vi "st_str Main.vi"() -> ()   [LabVIEW 2017]
doc: "This sample project is........"
uses:
  controls/st_str State.ctl
  controls/st_str Data.ctl
  controls/st_str UI References.ctl
  controls/st_str Graph Data.ctl
  <vilib>/Utility/miscctls.llb/LVAnnotationListTypeDef.ctl
  <vilib>/Utility/miscctls.llb/LVCursorListTypeDef.ctl
  controls/st_str User Specified Data.ctl
  controls/st_str HW Configuration.ctl
  controls/st_str Simulated Signal Type.ctl
  controls/st_str Analysis Configuration.ctl
  controls/st_str New Data Behavior.ctl
  st_voltmetr/subVIs/st_str Global.vi
  subVIs/st_str Settings Dialog(VIForIzm).vi
panel:
  in  "FirstActiveParam":bool
  out "АЧХ 2":cluster{dbl[], dbl[]}[](graph) caption="XY Graph - Light"
  in  "SetParametrsGen":bool
  out "Connect\nVoltmetr":bool
  in  "TypeGraph":T1(radio)
  in  "ResultTbl":string[][](table)
  out "Graph":waveform(dbl)[](graph)
  in  "Start":bool
  in  "View":enum16{"График", "Таблица"}(ring)
  in  "Open":bool
  in  "Delete":bool
  in  "Report":bool
  in  "Save":bool
  in  "Settings":bool
  in  "Snapshot":bool
  in  "Analyze":bool
  in  "Clear":bool
  in  "Exit":bool
  in  "Acquire":bool
  in  "Export":bool
  in  "Save Data":bool
  in  "Load Data":bool
  out "Status Bar":string
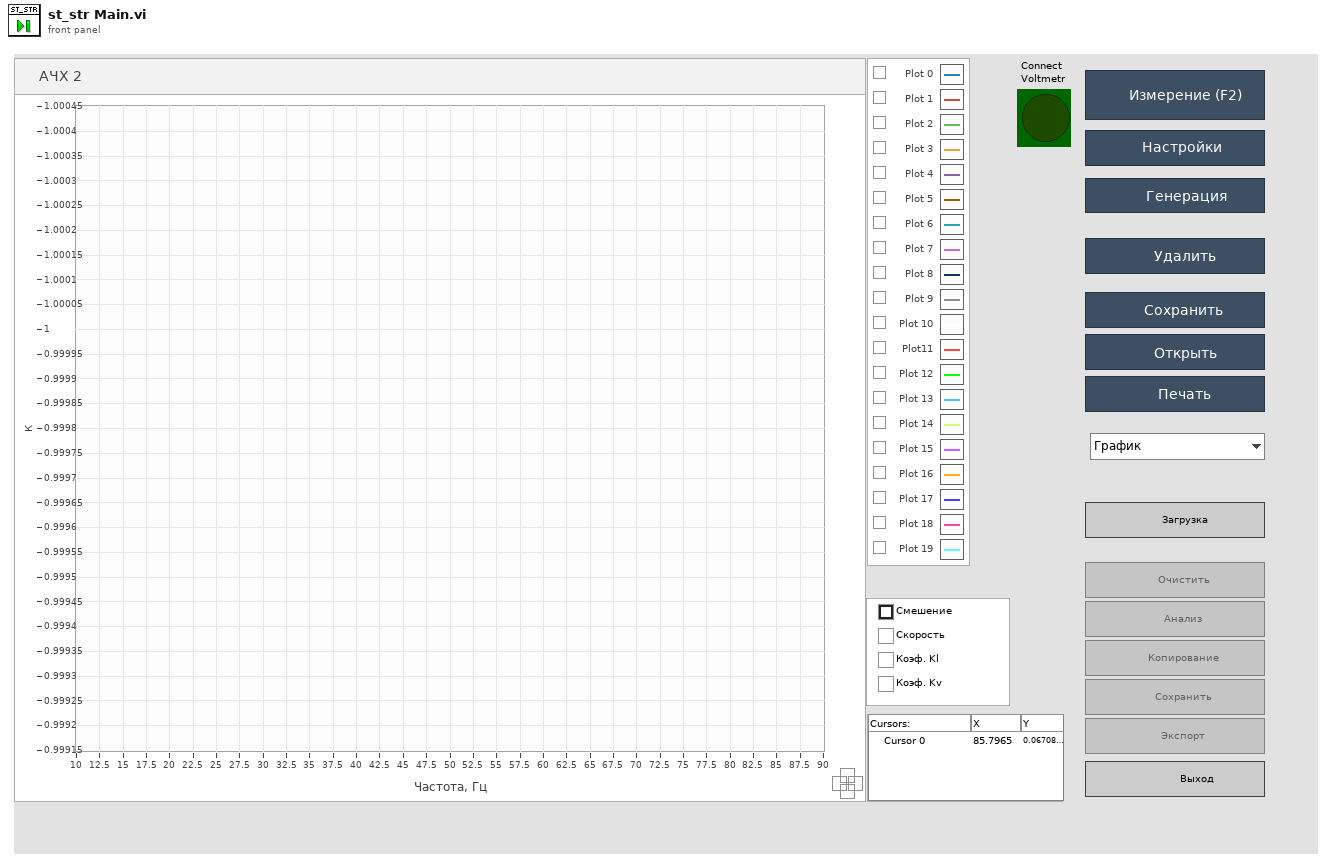
[diagram p1: front panel]
types:
  T1 = enum32{"Смешение", "Скорость", "Коэф. Kl", "Коэф. Kv"}
  T2 = typedef "st_str Data.ctl" = cluster{"UI References":T3, "Graph Data":T4, "User Specified":T7, "GenParametr":cluster{"UgenVrms":dbl, "Frequency 1,kHz":dbl, "dFreq, kHz":dbl, "Frequency 2,kHz":dbl, "WaitSignalGen":dbl}}
  T3 = typedef "st_str UI References.ctl" = cluster{"Exit Ref":refnum<vi>, "Save Ref":refnum<vi>, "Open Ref":refnum<vi>, "Export Ref":refnum<vi>, "Acquire Ref":refnum<vi>, "Configure Ref":refnum<vi>, "Graph Ref":refnum<vi>, "Clear Ref":refnum<vi>, "Analyze Ref":refnum<vi>, "Status Ref":refnum<vi>, "Snapshot Ref":refnum<vi>, "Tbl Ref":refnum<vi>, "XYGraph Ref":refnum<vi>}
  T4 = typedef "st_str Graph Data.ctl" = cluster{"Data":waveform(dbl)[], "Annotation List":T5, "Cursor List":T6, "Analysis Data":waveform(dbl)[], "XY graph":cluster{"X":dbl[], "Y":dbl[]}[]}
  T5 = typedef "LVAnnotationListTypeDef.ctl" = cluster{"Name":string, "Color":u32, "Style":u8, "Point Style":u8, "Name Visible":bool, "Allow Drag":bool, "Annotation Mode":u32, "Plot":i32, "Index":i32, "Position":cluster{"X":dbl, "Y":dbl}, "X Scale":u32, "Y Scale":u32, "Show Arrow":bool, "Lock Name":bool, "Plot Area":i32, "Label Offset":cluster{"X":dbl, "Y":dbl}}[]
  T6 = typedef "LVCursorListTypeDef.ctl" = cluster{"Name":string, "Color":u32, "Style":u8, "Point Style":u8, "Name Visible":bool, "Allow Drag":bool, "Cursor Mode":u32, "Plot":i32, "Index":i32, "Position":cluster{"X":dbl, "Y":dbl}, "X Scale":u32, "Y Scale":u32, "Watch Plots":i32[], "Watch All Plots":bool, "Plot Area":i32, "Label Offset":cluster{"X":dbl, "Y":dbl}}[]
  T7 = typedef "st_str User Specified Data.ctl" = cluster{"Hardware Configuration":T8, "Analysis Configuration":T10, "New Data Behavior":T11}
  T8 = typedef "st_str HW Configuration.ctl" = cluster{"HW Refnum <Replace Me>":string, "Signal Type <Replace Me>":T9}
  T9 = typedef "st_str Simulated Signal Type.ctl" = enum16{"Sine Wave", "Square Wave"}
  T10 = typedef "st_str Analysis Configuration.ctl" = cluster{"Statistics":bool}
  T11 = typedef "st_str New Data Behavior.ctl" = enum16{"Replace", "Overlay", "Append"}
  T12 = typedef "st_str State.ctl" = enum16{"View", "Initialize", "Wait for Event", "Update UI", "Configure", "Acquire", "Load Data", "Save Data", "Clear Data", "Export Data", "Analyze", "Copy Graph", "Exit", "Connecting"}
  T13 = cluster{"UgenVrms":dbl, "Frequency 1,kHz":dbl, "dFreq, kHz":dbl, "Frequency 2,kHz":dbl, "WaitSignalGen":dbl}
  T14 = typedef "st_str gen parametr.ctl" = cluster{"UgenVrms":dbl, "Frequency 1,kHz":dbl, "dFreq, kHz":dbl, "Frequency 2,kHz":dbl, "WaitSignalGen":dbl}
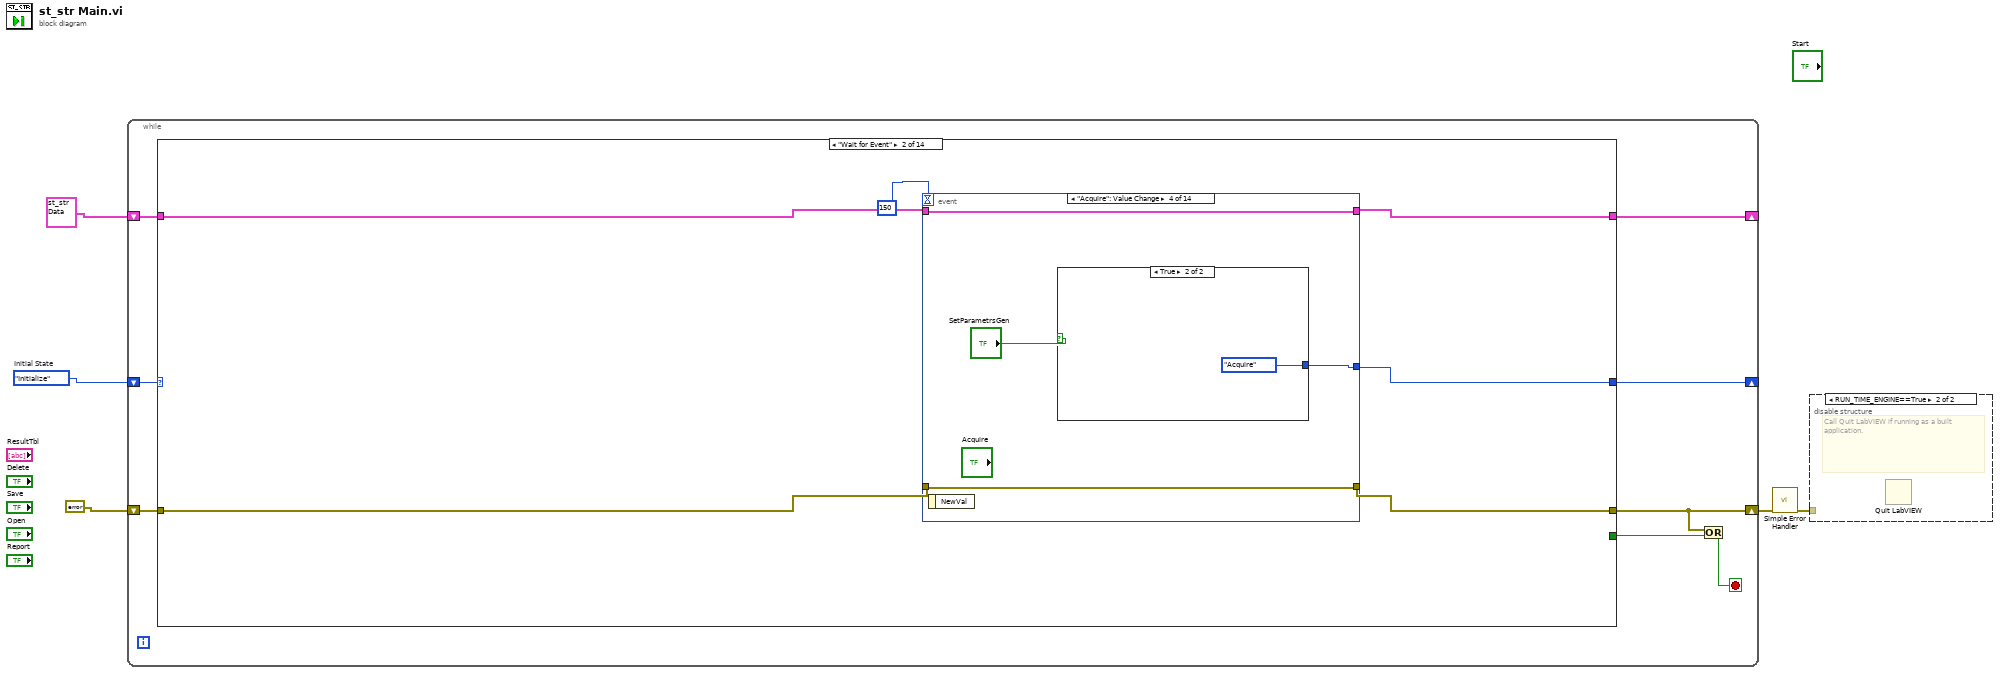
[diagram p0: block diagram]
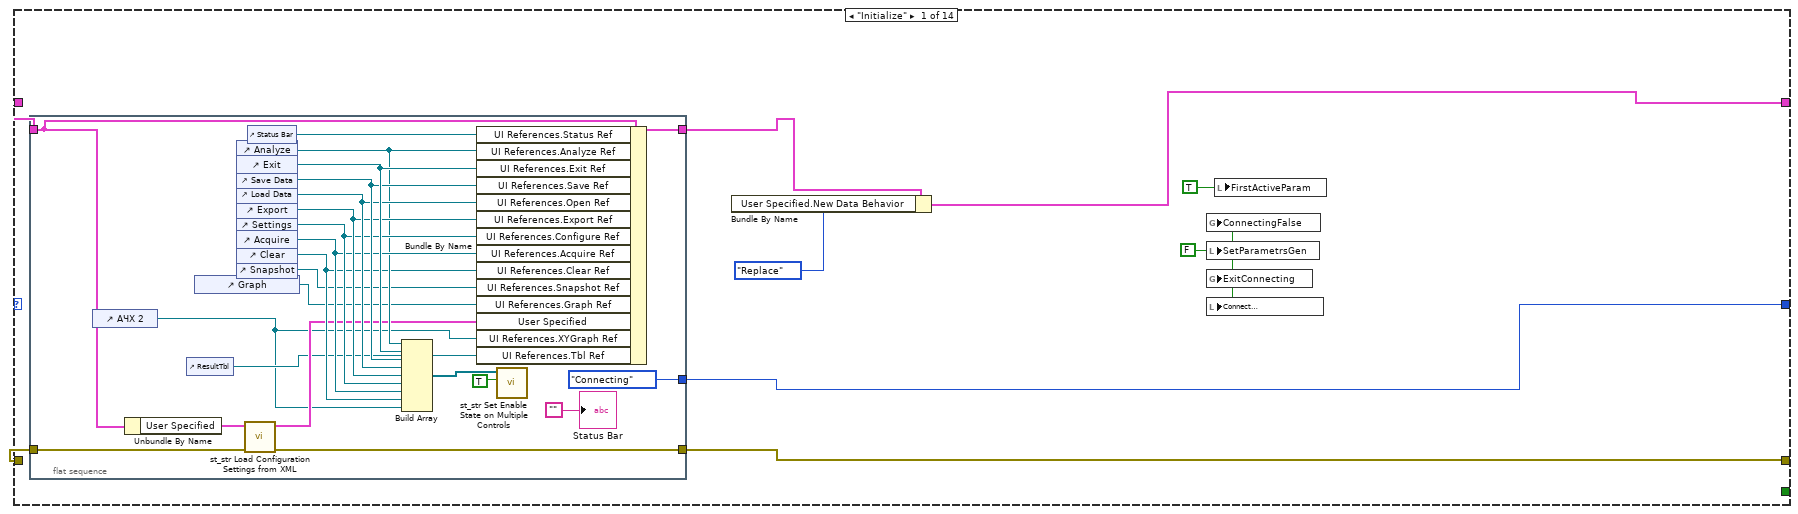
[diagram p3: hidden frame]
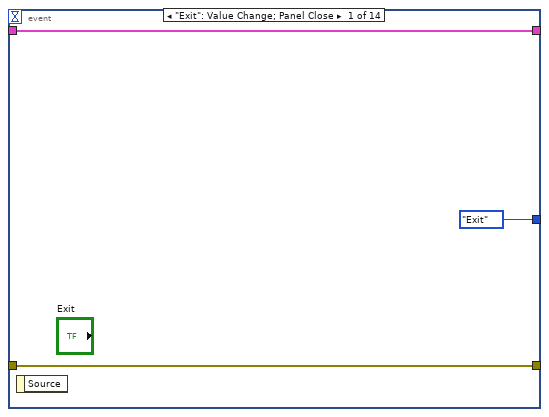
[diagram p4: hidden frame]
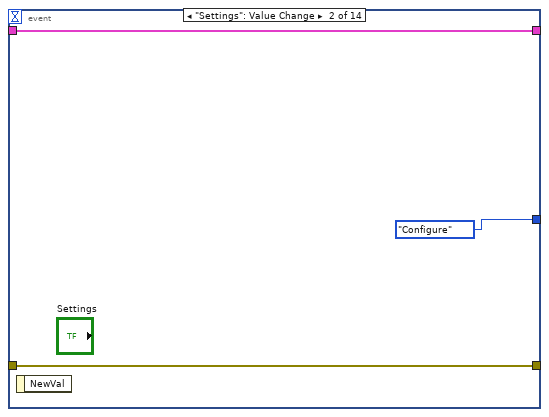
[diagram p5: hidden frame]
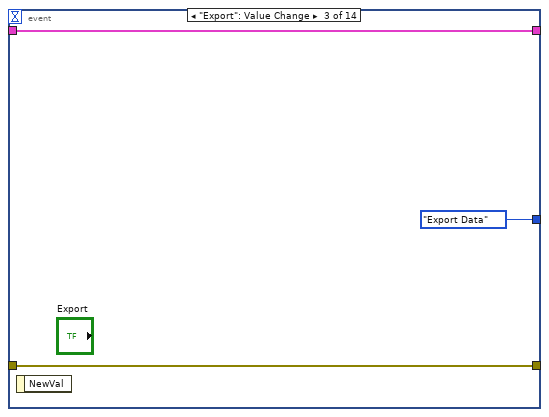
[diagram p6: hidden frame]
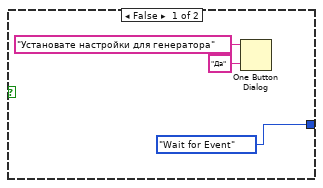
[diagram p7: hidden frame]
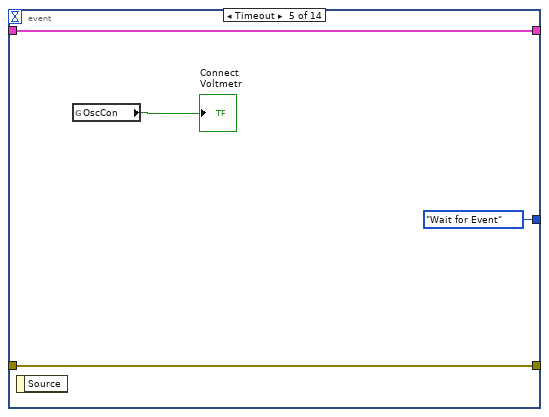
[diagram p8: hidden frame]
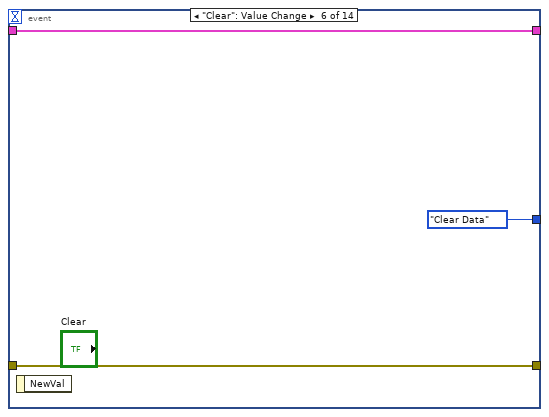
[diagram p9: hidden frame]
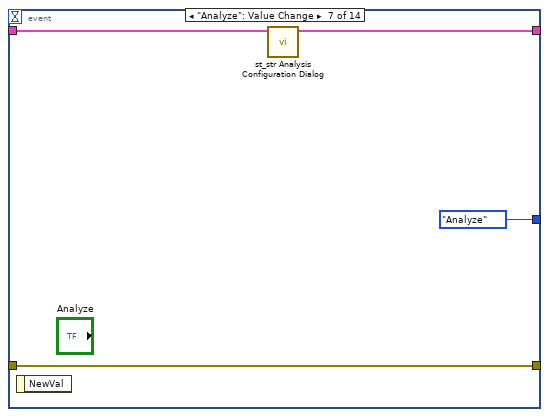
[diagram p10: hidden frame]
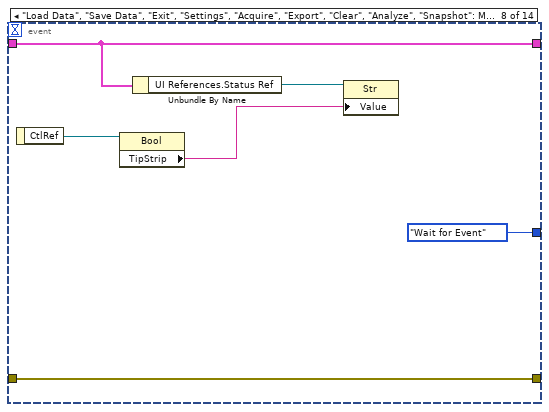
[diagram p11: hidden frame]
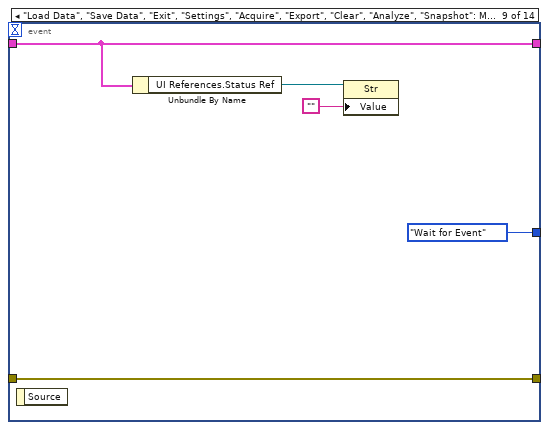
[diagram p12: hidden frame]
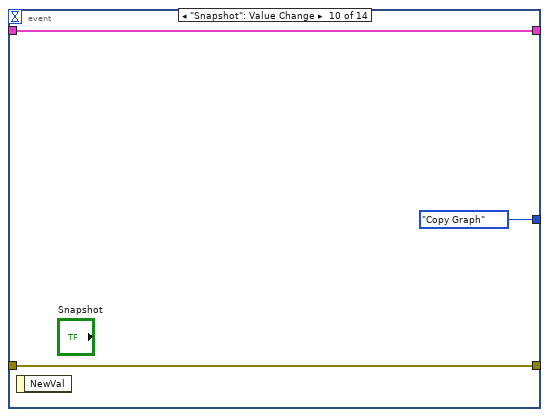
[diagram p13: hidden frame]
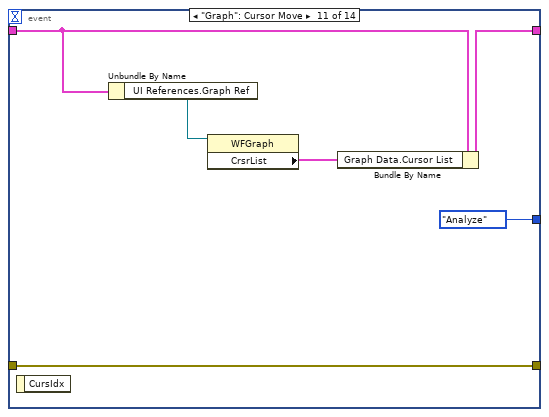
[diagram p14: hidden frame]
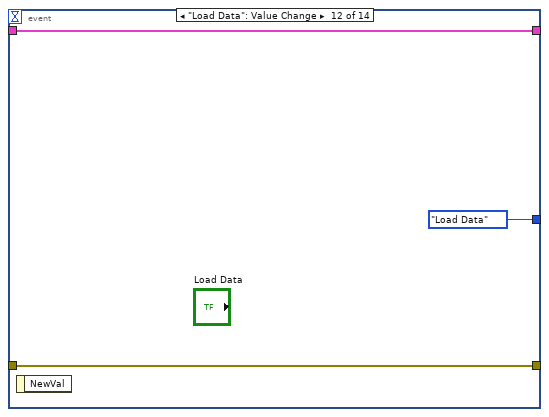
[diagram p15: hidden frame]
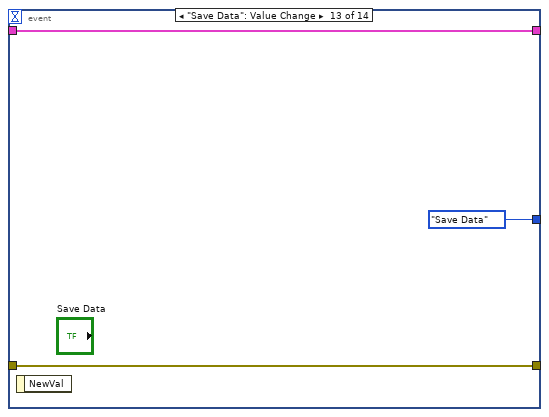
[diagram p16: hidden frame]
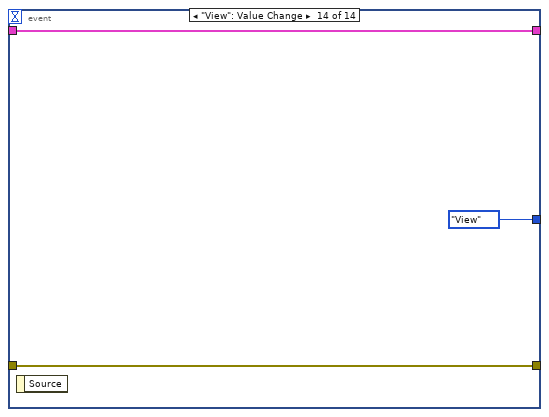
[diagram p17: hidden frame]
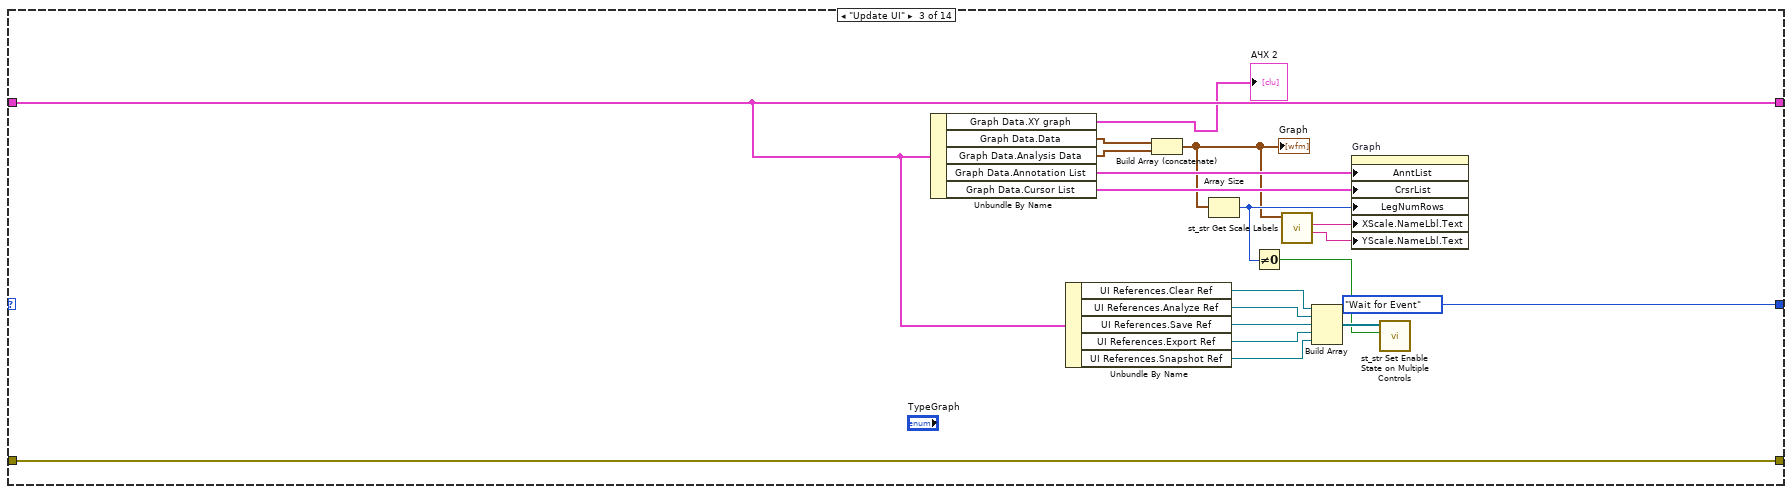
[diagram p18: hidden frame]
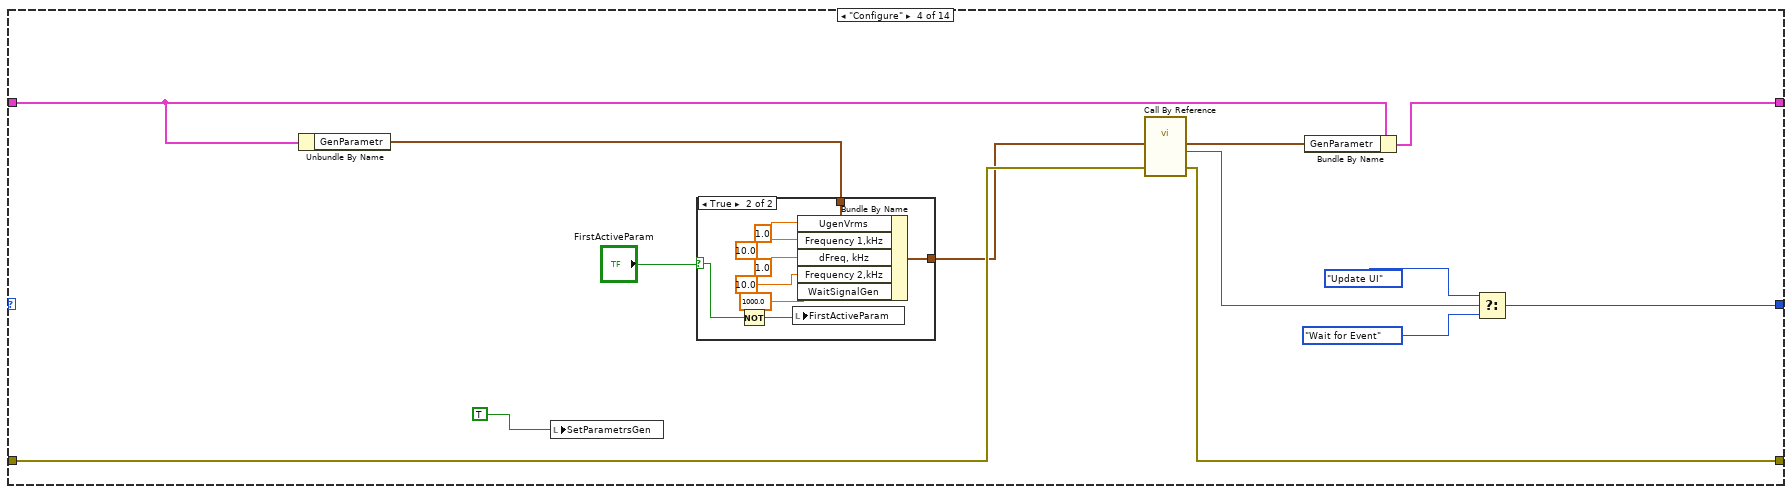
[diagram p19: hidden frame]
diagram:
  w5 = st_str_State."Initialize"  # Initial State
  n1 = while {
    shift-right: [w13] -> _
    shift-left: w5 -> [w6]
    shift-right: [w11] -> _
    shift-left: T2 {"UI References"={"Exit Ref"=refnum, "Save Ref"=refnum, "Open Ref"=refnum, "Export Ref"=refnum, "Acquire Ref"=refnum, "Configure Ref"=refnum, "Graph Ref"=refnum, "Clear Ref"=refnum, "Analyze Ref"=refnum, "Status Ref"=refnum, "Snapshot Ref"=refnum, "Tbl Ref"=refnum, "XYGraph Ref"=refnum}, "Graph Data"={"Data"=[], "Annotation List"=[], "Cursor List"=[], "Analysis Data"=[], "XY graph"=[]}, "User Specified"={"Hardware Configuration"={"HW Refnum <Replace Me>"="", "Signal Type <Replace Me>"=enum."Sine Wave"}, "Analysis Configuration"={"Statistics"=TRUE}, "New Data Behavior"=enum."Replace"}, "GenParametr"={"UgenVrms"=0.0, "Frequency 1,kHz"=0.0, "dFreq, kHz"=0.0, "Frequency 2,kHz"=0.0, "WaitSignalGen"=0.0}} ("Data") -> [w12]
    shift-right: [w7] -> w3
    shift-left: errorcluster {"status"=FALSE, "code"=0, "source"=""} ("error constant") -> [w10]
    stop <- w8 stop-if-true
    # "Finite Measurement State Machine"
    n2 = case shown="\"Wait for Event\"" w6 {
      tunnel: [w22 w51 st_str_State."Wait for Event" ("(Value Not Used)") w134 st_str_State."Update UI" ("Next State") st_str_State."Update UI" ("(Value Not Used)") st_str_State."Wait for Event" ("(Value Not Used)") st_str_State."Wait for Event" ("(Value Not Used)") st_str_State."Update UI" ("(Value Not Used)") st_str_State."Update UI" ("(Value Not Used)") st_str_State."Wait for Event" ("(Value Not Used)") w236 st_str_State."Update UI" ("(Value Not Used)") st_str_State."Update UI" ("(Value Not Used)")] -> w13
      tunnel: [_ _ _ _ _ _ _ _ _ _ _ w235 _ _] -> w9
      tunnel: w12 -> [w21 w50 w110 w140 w161 w182 w195 w207 w218 w221 w227 w233 w243 w260]
      tunnel: [w14 w49 w110 w139 w160 w176 w195 w207 w217 w221 w227 w233 w243 w260] -> w11
      tunnel: w10 -> [w20 w48 w127 w138 w155 w181 w197 w210 w220 w222 w226 w230 w247 w259]
      tunnel: [w19 w47 w127 w137 w158 w180 w193 w204 w220 w222 w225 w229 w247 w259] -> w7
      frame "Initialize" {
        w18 = FALSE ("Connect\nVoltmetr")
        n3 = flat-sequence {
          tunnel: [st_str_State."Connecting" ("Next State")] -> w22
          tunnel: [w44] -> w16
          tunnel: [w33] -> w19
          tunnel: w21 -> [w36]
          tunnel: w20 -> [w34]
          frame #0 {
            n4 = control-ref of="АЧХ 2"() -> (w23:refnum<vi>)
            n5 = Unbundle By Name(w36) -> ("User Specified"=w35:T7)
            n6 = control-ref of="ResultTbl"() -> (w24:refnum<vi>)
            n7 = control-ref of="Graph"() -> (w25:refnum<vi>)
            n8 = control-ref of="Analyze"() -> (w32:refnum<vi>)
            n9 = control-ref of="Exit"() -> (w43:refnum<vi>)
            n10 = control-ref of="Save Data"() -> (w42:refnum<vi>)
            n11 = control-ref of="Load Data"() -> (w41:refnum<vi>)
            n12 = control-ref of="Export"() -> (w40:refnum<vi>)
            n13 = control-ref of="Settings"() -> (w39:refnum<vi>)
            n14 = control-ref of="Acquire"() -> (w38:refnum<vi>)
            n15 = control-ref of="Clear"() -> (w30:refnum<vi>)
            n16 = control-ref of="Snapshot"() -> (w26:refnum<vi>)
            n17 = call "st_str Load Configuration Settings from XML.vi"("error in (no error)"=w34, "User Configuration in"=w35) -> ("error out"=w33:errorcluster, "User Configuration out"=w28:T7)  [unwired: 8 in]
            n18 = control-ref of="Status Bar"() -> (w31:refnum<vi>)
            n19 = Build Array(w32, w43, w42, w41, w40, w39, w38, w30, w23) -> (w37:refnum<vi>[])
            n20 = Bundle By Name(cluster=w36, "UI References.Status Ref"=w31, "UI References.Analyze Ref"=w32, "UI References.Exit Ref"=w43, "UI References.Save Ref"=w42, "UI References.Open Ref"=w41, "UI References.Export Ref"=w40, "UI References.Configure Ref"=w39, "UI References.Acquire Ref"=w38, "UI References.Clear Ref"=w30, "UI References.Snapshot Ref"=w26, "UI References.Graph Ref"=w25, "User Specified"=w28, "UI References.XYGraph Ref"=w23, "UI References.Tbl Ref"=w24) -> (w44:T2)
            n21 = call "st_str Set Enable State on Multiple Controls.vi"("Enable?"=TRUE, "Controls"=w37) -> ()  [unwired: 10 in]
            "Status Bar" <- "" ("Status Bar")
          }
        }
        n22 = Bundle By Name(cluster=w16, "User Specified.New Data Behavior"=st_str_New_Data_Behavior."Replace") -> (w14:T2)
        n23 = global write "st_str Global.vi" "ConnectingFalse"(w18) -> ()
        n24 = local write "SetParametrsGen"(w18) -> ()
        n25 = global write "st_str Global.vi" "ExitConnecting"(w18) -> ()
        n26 = local write "Connect\nVoltmetr"(w18) -> ()
        n27 = local write "FirstActiveParam"(TRUE ("FirstActiveParam")) -> ()
      }
      frame "Wait for Event" {
        n28 = event shown="[3] \"Acquire\": Value Change" {
          selector: _ -> [_ _ _ _ _ _ _ _ _ _ _ _ _ _]
          dyn-events: _ -> [_ _ _ _ _ _ _ _ _ _ _ _ _ _]
          timeout: 150 -> [_ _ _ _ _ _ _ _ _ _ _ _ _ _]
          tunnel: [st_str_State."Exit" ("Next State") st_str_State."Configure" ("Next State") st_str_State."Export Data" ("Next State") w62 st_str_State."Wait for Event" ("Next State") st_str_State."Clear Data" ("Next State") st_str_State."Analyze" ("Next State") st_str_State."Wait for Event" ("Next State") st_str_State."Wait for Event" ("Next State") st_str_State."Copy Graph" ("Next State") st_str_State."Analyze" ("Next State") st_str_State."Load Data" ("Next State") st_str_State."Save Data" ("Next State") st_str_State."View" ("Next State")] -> w51
          tunnel: w50 -> [w53 w57 w60 w64 w72 w75 w77 w83 w89 w93 w94 w101 w104 w108]
          tunnel: [w53 w57 w60 w64 w72 w75 w76 w83 w89 w93 w97 w101 w104 w108] -> w49
          tunnel: w48 -> [w52 w56 w59 w63 w71 w74 w79 w85 w90 w92 w99 w100 w103 w107]
          tunnel: [w52 w56 w59 w63 w71 w74 w79 w85 w90 w92 w99 w100 w103 w107] -> w47
          event "Exit": Value Change; Panel Close {
            n29 = event-data() -> ()  [unwired: 1 in, 1 out]
          }
          event "Settings": Value Change {
            n30 = event-data() -> ()  [unwired: 1 in, 1 out]
          }
          event "Export": Value Change {
            n31 = event-data() -> ()  [unwired: 1 in, 1 out]
          }
          event "Acquire": Value Change {
            n32 = event-data() -> ()  [unwired: 1 in, 1 out]
            n33 = case shown="True" "SetParametrsGen" {
              tunnel: [st_str_State."Wait for Event" ("Next State") st_str_State."Acquire" ("Next State")] -> w62
              frame False {
                n34 = One Button Dialog(message="Установате настройки для генератора", button name ("OK")="Да") -> ()  [unwired: 1 out]
              }
              frame True {
              }
            }
          }
          event Timeout {
            n35 = event-data() -> ()  [unwired: 1 in, 1 out]
            n36 = global read "st_str Global.vi" "OscCon"() -> (→"Connect\nVoltmetr":bool)
          }
          event "Clear": Value Change {
            n37 = event-data() -> ()  [unwired: 1 in, 1 out]
          }
          event "Analyze": Value Change {
            n38 = event-data() -> ()  [unwired: 1 in, 1 out]
            n39 = call "st_str Analysis Configuration Dialog.vi"("Data in"=w77) -> ("Data out"=w76:T2)  [unwired: 10 in]
          }
          event "Load Data", "Save Data", "Exit", "Settings", "Acquire", "Export", "Clear", "Analyze", "Snapshot": Mouse Enter {
            n40 = event-data() -> ("CtlRef"=w84:refnum<vi>)  [unwired: 1 in]
            n41 = property class="Bool"(reference=w84) -> ("TipStrip"=w81:string)  [unwired: 1 in, 2 out]
            n42 = Unbundle By Name(w83) -> ("UI References.Status Ref"=w82:refnum<vi>)
            n43 = property class="Str"(reference=w82, "Value"=w81) -> ()  [unwired: 1 in, 2 out]
          }
          event "Load Data", "Save Data", "Exit", "Settings", "Acquire", "Export", "Clear", "Analyze", "Snapshot": Mouse Leave {
            n44 = event-data() -> ()  [unwired: 1 in, 1 out]
            n45 = Unbundle By Name(w89) -> ("UI References.Status Ref"=w88:refnum<vi>)
            n46 = property class="Str"(reference=w88, "Value"="") -> ()  [unwired: 1 in, 2 out]
          }
          event "Snapshot": Value Change {
            n47 = event-data() -> ()  [unwired: 1 in, 1 out]
          }
          event "Graph": Cursor Move {
            n48 = event-data() -> ()  [unwired: 1 in, 1 out]
            n49 = Unbundle By Name(w94) -> ("UI References.Graph Ref"=w96:refnum<vi>)
            n50 = property class="WFGraph"(reference=w96) -> ("CrsrList"=w95:T6)  [unwired: 1 in, 2 out]
            n51 = Bundle By Name(cluster=w94, "Graph Data.Cursor List"=w95) -> (w97:T2)
          }
          event "Load Data": Value Change {
            n52 = event-data() -> ()  [unwired: 1 in, 1 out]
          }
          event "Save Data": Value Change {
            n53 = event-data() -> ()  [unwired: 1 in, 1 out]
          }
          event "View": Value Change {
            n54 = event-data() -> ()  [unwired: 1 in, 1 out]
          }
        }
      }
      frame "Update UI" {
        n55 = Unbundle By Name(w110) -> ("Graph Data.XY graph"=→"АЧХ 2":cluster{"X":dbl[], "Y":dbl[]}[], "Graph Data.Data"=w121:waveform(dbl)[], "Graph Data.Analysis Data"=w111:waveform(dbl)[], "Graph Data.Annotation List"=w125:T5, "Graph Data.Cursor List"=w122:T6)
        n56 = Unbundle By Name(w110) -> ("UI References.Clear Ref"=w117:refnum<vi>, "UI References.Analyze Ref"=w116:refnum<vi>, "UI References.Save Ref"=w124:refnum<vi>, "UI References.Export Ref"=w114:refnum<vi>, "UI References.Snapshot Ref"=w115:refnum<vi>)
        n57 = Build Array (concatenate)(w121, w111) -> (w119:waveform(dbl)[])
        "Graph" <- w119
        n58 = Array Size(array=w119) -> (size(s)=w120:i32)
        n59 = Not Equal To 0?(x=w120) -> (x != 0?=w118:bool)
        n60 = call "st_str Get Scale Labels.vi"("Array of Waveforms"=w119) -> ("Y Scale Label Text"=w112:string, "X Scale Label Text"=w113:string)  [unwired: 9 in]
        n61 = Build Array(w117, w116, w124, w114, w115) -> (w123:refnum<vi>[])
        n62 = property on="Graph" class="WFGraph (strict)"("AnntList"=w125, "CrsrList"=w122, "LegNumRows"=w120, "XScale.NameLbl.Text"=w113, "YScale.NameLbl.Text"=w112) -> ()  [unwired: 2 in, 2 out]
        n63 = call "st_str Set Enable State on Multiple Controls.vi"("Enable?"=w118, "Controls"=w123) -> ()  [unwired: 10 in]
      }
      frame "Configure" {
        n64 = Unbundle By Name(w140) -> ("GenParametr"=w131:T13)
        n65 = local write "SetParametrsGen"(TRUE ("SetParametrsGen")) -> ()
        n66 = case shown="True" "FirstActiveParam" {
          selector: "FirstActiveParam" -> [_ w142]
          tunnel: w131 -> [w141 w150]
          tunnel: [w141 w149] -> w130
          frame False {
          }
          frame True {
            n67 = Not(x=w142) -> (.not. x?=w143:bool)
            n68 = local write "FirstActiveParam"(w143) -> ()
            n69 = Bundle By Name(cluster=w150, "UgenVrms"=1.0, "Frequency 1,kHz"=10.0, "dFreq, kHz"=1.0, "Frequency 2,kHz"=10.0, "WaitSignalGen"=1000.0) -> (w149:T13)
          }
        }
        n70 = call-by-ref "?"("error in (no error)"=w138, "GenParametr"=w130) -> ("error out"=w137:errorcluster, "UI Refresh Needed?"=w136:bool, "GenParametr"=w132:T14)  [unwired: 9 in, 2 out]
        n71 = Bundle By Name(cluster=w140, "GenParametr"=w132) -> (w139:T2)
        n72 = Select(t=st_str_State."Update UI" ("Next State if true"), s=w136, f=st_str_State."Wait for Event" ("Next State if false")) -> (s? t:f=w134:T12)
      }
      frame "Acquire" {
        n73 = Unbundle By Name(w161) -> ("UI References.Status Ref"=w159:refnum<vi>, "GenParametr"=w154:T13)
        n74 = call "st_str Acquire Data from Hardware(forSubVi).vi"("error in (no error)"=w155, "GenParametr"=w154) -> ("error out"=w157:errorcluster, "AllParametrArray"=w156:dbl[][])  [unwired: 8 in]
        n75 = call "st_str RealiseArrayData(ViForIzm).vi"("error in (no error)"=w157, "AllParametrArray"=w156) -> ("error out"=w151:errorcluster, "appended array"=w152:cluster{dbl[], dbl[]}[], "Graph Data"=w153:waveform(dbl)[])  [unwired: 7 in]
        n76 = case shown="No Error" w151 {
          selector: w151 -> [w168 w172]
          tunnel: w161 -> [w167 w173]
          tunnel: [w170 w173] -> w160
          tunnel: [w169 _] -> w158
          tunnel: ["Data acquired." ("Data acquired") "Data not acquired." ("Data not acquired")] -> w162
          tunnel: w153 -> [w165 _]
          tunnel: w152 -> [w164 _]
          frame No Error {
            n77 = call "st_str Incorporate New Data.vi"("error in (no error)"=w168, "New Graph Data XY"=w164, "New Graph Data"=w165, "Data in"=w167) -> ("error out"=w169:errorcluster, "Data out"=w170:T2)  [unwired: 6 in]
          }
          frame Error {
            n78 = call <vilib>:"Simple Error Handler.vi"("error in (no error)"=w172) -> ()  [unwired: 4 in, 5 out]
          }
        }
        n79 = property class="Str"(reference=w159, "Value"=w162) -> ()  [unwired: 1 in, 2 out]
      }
      frame "Load Data" {
        # "Load Data - Loads data from a TDMS file and incorporates it with the existing data according to the user's preference."
        n80 = call "st_str Load Data.vi"("error in (no error)"=w181) -> ("error out"=w178:errorcluster, "New Graph Data"=w175:waveform(dbl)[])  [unwired: 9 in]
        n81 = case shown="No Error" w178 {
          selector: w178 -> [w185 w190]
          tunnel: w182 -> [w184 w191]
          tunnel: [w188 w191] -> w176
          tunnel: [w187 _] -> w180
          tunnel: w175 -> [w186 _]
          tunnel: ["Data loaded." ("Data loaded") "Data not loaded." ("Data not loaded")] -> w177
          frame No Error {
            n82 = call "st_str Incorporate New Data.vi"("error in (no error)"=w185, "New Graph Data"=w186, "Data in"=w184) -> ("error out"=w187:errorcluster, "Data out"=w188:T2)  [unwired: 7 in]
          }
          frame Error {
            n83 = call <vilib>:"Simple Error Handler.vi"("error in (no error)"=w190) -> ()  [unwired: 4 in, 5 out]
          }
        }
        n84 = Unbundle By Name(w176) -> ("UI References.Status Ref"=w174:refnum<vi>)
        n85 = property class="Str"(reference=w174, "Value"=w177) -> ()  [unwired: 1 in, 2 out]
      }
      frame "Save Data" {
        # "Save Data - Saves the existing measurement data to a TDMS file."
        n86 = Unbundle By Name(w195) -> ("UI References.Status Ref"=w194:refnum<vi>, "Graph Data.Data"=w198:waveform(dbl)[])
        n87 = call "st_str Save Data.vi"("error in (no error)"=w197, "Data"=w198) -> ("error out"=w196:errorcluster)  [unwired: 9 in]
        n88 = case shown="No Error" w196 {
          selector: w196 -> [w200 w203]
          tunnel: ["Data saved." ("Data saved") "Data not saved." ("Data not saved")] -> w192
          tunnel: [w200 _] -> w193
          frame No Error {
          }
          frame Error {
            n89 = call <vilib>:"Simple Error Handler.vi"("error in (no error)"=w203) -> ()  [unwired: 4 in, 5 out]
          }
        }
        n90 = property class="Str"(reference=w194, "Value"=w192) -> ()  [unwired: 1 in, 2 out]
      }
      frame "Export Data" {
        # "Export Data - Exports the currently loaded measurement and analysis data to a text file that can be imported into a spreadsheet or other application."
        n91 = Unbundle By Name(w207) -> ("UI References.Status Ref"=w205:refnum<vi>, "Graph Data"=w206:T4)
        n92 = call "st_str Export Data.vi"("error in (no error)"=w210, "Graph Data"=w206) -> ("error out"=w208:errorcluster)  [unwired: 9 in]
        n93 = case shown="No Error" w208 {
          selector: w208 -> [w212 w215]
          tunnel: ["Data exported." ("Data exported") "Data not exported." ("Data not exported")] -> w209
          tunnel: [w212 _] -> w204
          frame No Error {
          }
          frame Error {
            n94 = call <vilib>:"Simple Error Handler.vi"("error in (no error)"=w215) -> ()  [unwired: 4 in, 5 out]
          }
        }
        n95 = property class="Str"(reference=w205, "Value"=w209) -> ()  [unwired: 1 in, 2 out]
      }
      frame "Clear Data" {
        # "Clear Data - Clears the data currently in the graph."
        n96 = Bundle By Name(cluster=w218, "Graph Data"=T4 {"Data"=[], "Annotation List"=[], "Cursor List"=[], "Analysis Data"=[], "XY graph"=[]} ("Graph")) -> (w217:T2)
      }
      frame "Analyze" {
        # "#CodeRecommended - Add your own signal analysis here."
        # "Analyze - Analyzes the measurement data."
        n97 = Unbundle By Name(w221) -> ("Graph Data"=w223:T4)
        n98 = call "st_str Statistical Analysis.vi"("Graph Data In"=w223) -> ()  [unwired: 9 in, 2 out]
      }
      frame "Copy Graph" {
        # "Copy Graph - Places an image of the graph on the clipboard for pasting into reports or emails."
        n99 = call "st_str Copy Graph to Clipboard.vi"("error in (no error)"=w226, "Graph Data"=w227) -> ("error out"=w225:errorcluster)  [unwired: 9 in]
      }
      frame "Exit" {
        w235 = TRUE  # Stop Loop?
        w236 = st_str_State."Exit"  # (Value Not Used)
        # "Exit - Saves the user's settings to an XML file and stops execution."
        n100 = Unbundle By Name(w233) -> ("UI References.Status Ref"=w231:refnum<vi>, "User Specified"=w234:T7)
        n101 = flat-sequence {
          frame #0 {
            n102 = global write "st_str Global.vi" "WorkVoltmetr"(FALSE) -> ()
          }
          frame #1 {
            n103 = Wait (ms)(milliseconds to wait=u32 2000) -> ()  [unwired: 1 out]
          }
          frame #2 {
            n104 = vi-ref "st_voltmetr.vi"() -> (w239:refnum<vi>)
            n105 = call "CloseVi (SubVI).vi"("VI in"=w239) -> ()  [unwired: 11 in]
          }
        }
        n106 = call "st_str Save Configuration Settings to XML.vi"("error in (no error)"=w230, "User Configuration"=w234) -> ("error out"=w229:errorcluster)  [unwired: 9 in]
        n107 = property class="Str"(reference=w231, "Value"="Application exit." ("Stopped")) -> ()  [unwired: 1 in, 2 out]
      }
      frame "View" {
        n108 = case shown="\"Таблица\"" "View" {
          tunnel: w243 -> [w252 w257]
          tunnel: [w250 w256] -> w241
          tunnel: [w249 w255] -> w240
          frame "График", Default {
            n109 = Unbundle By Name(w252) -> ("UI References.Tbl Ref"=w251:refnum<vi>, "UI References.XYGraph Ref"=w248:refnum<vi>)
            n110 = Build Array(w251) -> (w250:refnum<vi>[])
            n111 = Build Array(w248) -> (w249:refnum<vi>[])
          }
          frame "Таблица" {
            n112 = Unbundle By Name(w257) -> ("UI References.Tbl Ref"=w253:refnum<vi>, "UI References.XYGraph Ref"=w254:refnum<vi>)
            n113 = Build Array(w254) -> (w256:refnum<vi>[])
            n114 = Build Array(w253) -> (w255:refnum<vi>[])
          }
        }
        n115 = call "st_str Set Visable on Multiple Controls.vi"("Visable?"=TRUE ("Enable?"), "Controls"=w240) -> ()  [unwired: 10 in]
        n116 = call "st_str Set Visable on Multiple Controls.vi"("Visable?"=FALSE ("Enable?"), "Controls"=w241) -> ()  [unwired: 10 in]
      }
      frame "Connecting" {
        n117 = flat-sequence {
          frame #0 {
            n118 = vi-ref "st_voltmetr.vi"() -> (w261:refnum<vi>)
            n119 = call "OpenAndRunVi (SubVI).vi"("VI in"=w261) -> ()  [unwired: 11 in]
          }
          frame #1 {
            n120 = vi-ref "Connecting(Sub VI).vi"() -> (w265:refnum<vi>)
            n121 = call "OpenAndRunVi (SubVI) — with saw.vi"("VI in"=w265) -> ()  [unwired: 11 in]
            n122 = Tick Count (ms)() -> (millisecond timer value=w264:u32)
            n123 = Add(x=w264, y=u32 80000) -> (x+y=w262:u32)
            n124 = while {
              tunnel: w262 -> [w271]
              stop <- w270 stop-if-true
              n125 = global read "st_str Global.vi" "ConnectingFalse"() -> (w267:bool)
              n126 = global read "st_str Global.vi" "ExitConnecting"() -> (w266:bool)
              n127 = Tick Count (ms)() -> (millisecond timer value=w272:u32)
              n128 = global read "st_str Global.vi" "OscCon"() -> (w268:bool)
              n129 = Greater?(x=w272, y=w271) -> (0:w269:bool)
              n130 = Compound Arithmetic op=OR(w269, w267, w268, w266) -> (w270:bool)
            }
          }
          frame #2 {
            n131 = vi-ref "st_voltmetr.vi"() -> (w273:refnum<vi>)
            n132 = call "CloseVi (SubVI).vi"("VI in"=w273) -> ()  [unwired: 11 in]
          }
          frame #3 {
            n133 = Wait (ms)(milliseconds to wait=u32 1000) -> ()  [unwired: 1 out]
          }
          frame #4 {
            n134 = vi-ref "Connecting(Sub VI).vi"() -> (w275:refnum<vi>)
            n135 = call "CloseVi (SubVI).vi"("VI in"=w275) -> ()  [unwired: 11 in]
          }
        }
      }
    }
    n136 = Or(x=w7, y=w9) -> (x .or. y?=w8:bool)
  }
  n137 = call <vilib>:"Simple Error Handler.vi"("error in (no error)"=w3) -> ("error out"=w1:errorcluster)  [unwired: 4 in, 4 out]
  n138 = disable-structure shown="RUN_TIME_ENGINE==True" {
    disable-tunnel: w1 -> [_ _]
    frame condition #0 (active) {
    }
    frame condition #1 {
      # "Call Quit LabVIEW if running as a built application."
      n139 = Quit LabVIEW() -> ()  [unwired: 1 in]
    }
  }
